vi "Disconnect.vi"(8 "error in":errorcluster, 11 "BKPrecision in":refnum<class "9115AT.lvclass">) -> (0 "error out":errorcluster, 3 "BKPrecision out":refnum<class "9115AT.lvclass">)   [LabVIEW 2018, in "9115AT.lvlib" / "9115AT.lvclass"]
uses:
  9115AT.lvclass
  <instrlib>/BK Precision 911X Series/BK Precision 911X Series.lvlib
  builds/Power_Supply.lvlibp/Power Supply.lvclass
  C:/Users/Ron.Dexter.LUMINARTECH/Desktop/builds/Power_Supply.lvlibp/Power Supply.lvclass
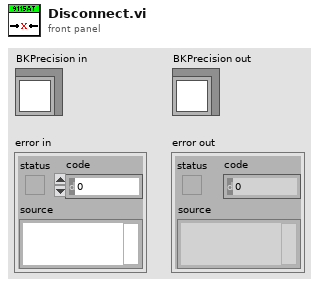
[diagram p1: front panel]
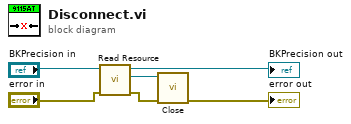
[diagram p0: block diagram]
diagram:
  n1 = call "Read Resource.vi"("error in"="error in", "Power Supply in"="BKPrecision in") -> ("error out"=w4:errorcluster, "Resource"=w3:refnum<visa-resource-name>, "Power Supply out"=→"BKPrecision out":refnum<class "9115AT.lvclass">)  [unwired: 7 in]
  n2 = call <instrlib>:"Close.vi"("error in (no error)"=w4, "VISA resource name"=w3) -> ("error out"=→"error out":errorcluster)  [unwired: 9 in]
